vi "HFRR ADV v09.vi"() -> ()   [LabVIEW 2025] (continued)
            n3661 = property on="SPEED OUT:" class="DigNum (strict)"("Caption.Text"=w4886) -> ()  [unwired: 2 in, 2 out]
            n3662 = property on="AIR TEMPERATURE :" class="DigNum (strict)"("Caption.Text"=w4885) -> ()  [unwired: 2 in, 2 out]
            n3663 = property on="HUMIDITY:" class="DigNum (strict)"("Caption.Text"=w4884) -> ()  [unwired: 2 in, 2 out]
            n3664 = property on="EDIT" class="Bool (strict)"("Boolean Text.Text"=w4883) -> ()  [unwired: 2 in, 2 out]
            n3665 = local read "S 79"() -> (w4870:string)
            n3666 = property on="Stroke" class="DigNum (strict)"("Caption.Text"=w4870) -> ()  [unwired: 2 in, 2 out]
          }
          frame #2 {
          }
        }
        n3667 = local write "Lan flag"(10.0 ("Lan flag")) -> ()
      }
      frame Enabled {
      }
    }
    n3668 = Wait (ms)(milliseconds to wait=u32 2000) -> ()  [unwired: 1 out]
    n3669 = local read "Quit"() -> (w4672:bool)
  }
  n3670 = disable-structure shown="Disabled" {
    frame Disabled {
      n3671 = while {
        tunnel: [w4901] -> _
        i -> [w4901]
        stop <- w4900 continue-if-true
        n3672 = Wait (ms)(milliseconds to wait=u32 50) -> ()  [unwired: 1 out]
        n3673 = stacked-sequence {
          frame #0 {
            # "Controls Text color"
            # "Controls BG color"
            n3674 = property on="FILE" class="Str"("Text.Text Colors:Text Color"="SC  Text") -> ()  [unwired: 2 in, 2 out]
            n3675 = property on="Fuel Discription :" class="Str"("Text.Text Colors:Text Color"="SC  Text") -> ()  [unwired: 2 in, 2 out]
            n3676 = property on="tested by" class="Str"("Text.Text Colors:Text Color"="SC  Text") -> ()  [unwired: 2 in, 2 out]
            n3677 = property on="Remarks :" class="Str"("Text.Text Colors:Text Color"="SC  Text") -> ()  [unwired: 2 in, 2 out]
            n3678 = property class="DigNum (strict)"("Numeric Text.Text Colors:BG Color"="NC BG") -> ()  [unwired: 2 in, 2 out]
            n3679 = property class="DigNum (strict)"("Numeric Text.Text Colors:BG Color"="NC BG") -> ()  [unwired: 2 in, 2 out]
            n3680 = property class="DigNum (strict)"("Numeric Text.Text Colors:BG Color"="NC BG") -> ()  [unwired: 2 in, 2 out]
            n3681 = property class="DigNum (strict)"("Numeric Text.Text Colors:BG Color"="NC BG") -> ()  [unwired: 2 in, 2 out]
            n3682 = property class="DigNum (strict)"("Numeric Text.Text Colors:BG Color"="NC BG") -> ()  [unwired: 2 in, 2 out]
            n3683 = property class="DigNum (strict)"("Numeric Text.Text Colors:BG Color"="NC BG") -> ()  [unwired: 2 in, 2 out]
            n3684 = property class="DigNum (strict)"("Numeric Text.Text Colors:BG Color"="NC BG") -> ()  [unwired: 2 in, 2 out]
            n3685 = property class="DigNum (strict)"("Numeric Text.Text Colors:BG Color"="NC BG") -> ()  [unwired: 2 in, 2 out]
            n3686 = property class="DigNum (strict)"("Numeric Text.Text Colors:BG Color"="NC BG") -> ()  [unwired: 2 in, 2 out]
            n3687 = property class="DigNum (strict)"("Numeric Text.Text Colors:BG Color"="NC BG") -> ()  [unwired: 2 in, 2 out]
            n3688 = property class="DigNum (strict)"("Numeric Text.Text Colors:BG Color"="NC BG") -> ()  [unwired: 2 in, 2 out]
            n3689 = property class="DigNum (strict)"("Numeric Text.Text Colors:BG Color"="NC BG") -> ()  [unwired: 2 in, 2 out]
            n3690 = property on="FILE" class="Str"("Text.Text Colors:BG Color"="SC BG 3") -> ()  [unwired: 2 in, 2 out]
            n3691 = property on="Fuel Discription :" class="Str"("Text.Text Colors:BG Color"="SC BG 3") -> ()  [unwired: 2 in, 2 out]
            n3692 = property on="tested by" class="Str"("Text.Text Colors:BG Color"="SC BG 3") -> ()  [unwired: 2 in, 2 out]
            n3693 = property on="Remarks :" class="Str"("Text.Text Colors:BG Color"="SC BG 3") -> ()  [unwired: 2 in, 2 out]
            n3694 = property class="DigNum (strict)"("Numeric Text.Text Colors:Text Color"="NC Text") -> ()  [unwired: 2 in, 2 out]
            n3695 = property class="DigNum (strict)"("Numeric Text.Text Colors:Text Color"="NC Text") -> ()  [unwired: 2 in, 2 out]
            n3696 = property class="DigNum (strict)"("Numeric Text.Text Colors:Text Color"="NC Text") -> ()  [unwired: 2 in, 2 out]
            n3697 = property class="DigNum (strict)"("Numeric Text.Text Colors:Text Color"="NC Text") -> ()  [unwired: 2 in, 2 out]
            n3698 = property class="DigNum (strict)"("Numeric Text.Text Colors:Text Color"="NC Text") -> ()  [unwired: 2 in, 2 out]
            n3699 = property class="DigNum (strict)"("Numeric Text.Text Colors:Text Color"="NC Text") -> ()  [unwired: 2 in, 2 out]
            n3700 = property class="DigNum (strict)"("Numeric Text.Text Colors:Text Color"="NC Text") -> ()  [unwired: 2 in, 2 out]
            n3701 = property class="DigNum (strict)"("Numeric Text.Text Colors:Text Color"="NC Text") -> ()  [unwired: 2 in, 2 out]
            n3702 = property class="DigNum (strict)"("Numeric Text.Text Colors:Text Color"="NC Text") -> ()  [unwired: 2 in, 2 out]
            n3703 = property class="DigNum (strict)"("Numeric Text.Text Colors:Text Color"="NC Text") -> ()  [unwired: 2 in, 2 out]
            n3704 = property class="DigNum (strict)"("Numeric Text.Text Colors:Text Color"="NC Text") -> ()  [unwired: 2 in, 2 out]
            n3705 = property class="DigNum (strict)"("Numeric Text.Text Colors:Text Color"="NC Text") -> ()  [unwired: 2 in, 2 out]
            n3706 = property class="DigNum (strict)"("Numeric Text.Text Colors:Text Color"="NI Text  2") -> ()  [unwired: 2 in, 2 out]
            n3707 = property class="DigNum (strict)"("Numeric Text.Text Colors:Text Color"="NI Text  2") -> ()  [unwired: 2 in, 2 out]
            n3708 = property class="DigNum (strict)"("Numeric Text.Text Colors:Text Color"="NI Text  2") -> ()  [unwired: 2 in, 2 out]
            n3709 = property class="DigNum (strict)"("Numeric Text.Text Colors:Text Color"="NI Text  2") -> ()  [unwired: 2 in, 2 out]
            n3710 = property class="DigNum (strict)"("Numeric Text.Text Colors:Text Color"="NI Text  2") -> ()  [unwired: 2 in, 2 out]
            n3711 = property class="DigNum (strict)"("Numeric Text.Text Colors:Text Color"="NI Text  2") -> ()  [unwired: 2 in, 2 out]
            n3712 = property class="DigNum (strict)"("Numeric Text.Text Colors:Text Color"="NI Text  2") -> ()  [unwired: 2 in, 2 out]
            n3713 = property class="DigNum (strict)"("Numeric Text.Text Colors:Text Color"="NI Text  2") -> ()  [unwired: 2 in, 2 out]
            n3714 = property class="DigNum (strict)"("Numeric Text.Text Colors:Text Color"="NI Text  2") -> ()  [unwired: 2 in, 2 out]
            n3715 = property class="DigNum (strict)"("Numeric Text.Text Colors:Text Color"="NI Text  2") -> ()  [unwired: 2 in, 2 out]
            n3716 = property class="DigNum (strict)"("Numeric Text.Text Colors:Text Color"="NI Text  2") -> ()  [unwired: 2 in, 2 out]
            n3717 = property class="DigNum (strict)"("Numeric Text.Text Colors:Text Color"="NI Text  2") -> ()  [unwired: 2 in, 2 out]
            n3718 = property class="DigNum (strict)"("Numeric Text.Text Colors:Text Color"="NI Text  2") -> ()  [unwired: 2 in, 2 out]
            n3719 = property class="DigNum (strict)"("Numeric Text.Text Colors:Text Color"="NI Text  2") -> ()  [unwired: 2 in, 2 out]
            n3720 = property class="DigNum (strict)"("Numeric Text.Text Colors:Text Color"="NI Text  2") -> ()  [unwired: 2 in, 2 out]
            n3721 = property class="DigNum (strict)"("Numeric Text.Text Colors:Text Color"="NI Text  2") -> ()  [unwired: 2 in, 2 out]
            n3722 = property on="Coefficient Of Friction" class="XYGraph (strict)"("Plot Area:Colors:FG Color"="GFG  2", "Plot Area:Colors:BG Color"="GBG   2") -> ()  [unwired: 2 in, 2 out]
            n3723 = property on="Humidity ( %RH )" class="XYGraph (strict)"("Plot Area:Colors:FG Color"="GFG  2", "Plot Area:Colors:BG Color"="GBG   2") -> ()  [unwired: 2 in, 2 out]
            n3724 = property on="Air Temperature  ( °C )" class="XYGraph (strict)"("Plot Area:Colors:FG Color"="GFG  2", "Plot Area:Colors:BG Color"="GBG   2") -> ()  [unwired: 2 in, 2 out]
            n3725 = property on="Sample Temperature ( °C )" class="XYGraph (strict)"("Plot Area:Colors:FG Color"="GFG  2", "Plot Area:Colors:BG Color"="GBG   2") -> ()  [unwired: 2 in, 2 out]
            n3726 = property class="DigNum (strict)"("Numeric Text.Text Colors:BG Color"="NI BG 2") -> ()  [unwired: 2 in, 2 out]
            n3727 = property class="DigNum (strict)"("Numeric Text.Text Colors:BG Color"="NI BG 2") -> ()  [unwired: 2 in, 2 out]
            n3728 = property class="DigNum (strict)"("Numeric Text.Text Colors:BG Color"="NI BG 2") -> ()  [unwired: 2 in, 2 out]
            n3729 = property class="DigNum (strict)"("Numeric Text.Text Colors:BG Color"="NI BG 2") -> ()  [unwired: 2 in, 2 out]
            n3730 = property class="DigNum (strict)"("Numeric Text.Text Colors:BG Color"="NI BG 2") -> ()  [unwired: 2 in, 2 out]
            n3731 = property class="DigNum (strict)"("Numeric Text.Text Colors:BG Color"="NI BG 2") -> ()  [unwired: 2 in, 2 out]
            n3732 = property class="DigNum (strict)"("Numeric Text.Text Colors:BG Color"="NI BG 2") -> ()  [unwired: 2 in, 2 out]
            n3733 = property class="DigNum (strict)"("Numeric Text.Text Colors:BG Color"="NI BG 2") -> ()  [unwired: 2 in, 2 out]
            n3734 = property class="DigNum (strict)"("Numeric Text.Text Colors:BG Color"="NI BG 2") -> ()  [unwired: 2 in, 2 out]
            n3735 = property class="DigNum (strict)"("Numeric Text.Text Colors:BG Color"="NI BG 2") -> ()  [unwired: 2 in, 2 out]
            n3736 = property class="DigNum (strict)"("Numeric Text.Text Colors:BG Color"="NI BG 2") -> ()  [unwired: 2 in, 2 out]
            n3737 = property class="DigNum (strict)"("Numeric Text.Text Colors:BG Color"="NI BG 2") -> ()  [unwired: 2 in, 2 out]
            n3738 = property class="DigNum (strict)"("Numeric Text.Text Colors:BG Color"="NI BG 2") -> ()  [unwired: 2 in, 2 out]
            n3739 = property class="DigNum (strict)"("Numeric Text.Text Colors:BG Color"="NI BG 2") -> ()  [unwired: 2 in, 2 out]
            n3740 = property class="DigNum (strict)"("Numeric Text.Text Colors:BG Color"="NI BG 2") -> ()  [unwired: 2 in, 2 out]
            n3741 = property class="DigNum (strict)"("Numeric Text.Text Colors:BG Color"="NI BG 2") -> ()  [unwired: 2 in, 2 out]
            n3742 = property class="Bool"("Colors [4]"="Boolean BC T & BG") -> ()  [unwired: 2 in, 2 out]
            n3743 = property on="Save & Continue" class="Bool (strict)"("Colors [4]"="Boolean BC T & BG") -> ()  [unwired: 2 in, 2 out]
            n3744 = property on="Heater Button" class="Bool (strict)"("Colors [4]"="Boolean BC T & BG") -> ()  [unwired: 2 in, 2 out]
            n3745 = property class="Bool"("Colors [4]"="Boolean BC T & BG") -> ()  [unwired: 2 in, 2 out]
            n3746 = property on="Humidity" class="Bool (strict)"("Colors [4]"="Boolean BC T & BG") -> ()  [unwired: 2 in, 2 out]
            n3747 = property class="Bool (strict)"("Colors [4]"="Boolean BC T & BG") -> ()  [unwired: 2 in, 2 out]
            n3748 = property on="RUN" class="Bool (strict)"("Colors [4]"="Boolean BC T & BG") -> ()  [unwired: 2 in, 2 out]
            n3749 = property on="trip1 8" class="Bool (strict)"("Colors [4]"="Boolean BC T & BG") -> ()  [unwired: 2 in, 2 out]
            n3750 = property class="Bool"("Colors [4]"="Boolean BC T & BG") -> ()  [unwired: 2 in, 2 out]
            n3751 = property class="Bool (strict)"("Colors [4]"="Boolean BC T & BG") -> ()  [unwired: 2 in, 2 out]
            n3752 = property on="OPEN 1" class="Bool (strict)"("Colors [4]"="Boolean BC T & BG 2") -> ()  [unwired: 2 in, 2 out]
            n3753 = property on="OPEN 2" class="Bool (strict)"("Colors [4]"="Boolean BC T & BG 2") -> ()  [unwired: 2 in, 2 out]
            n3754 = property on="OPEN 3" class="Bool (strict)"("Colors [4]"="Boolean BC T & BG 2") -> ()  [unwired: 2 in, 2 out]
            n3755 = property on="OPEN 4" class="Bool (strict)"("Colors [4]"="Boolean BC T & BG 2") -> ()  [unwired: 2 in, 2 out]
            n3756 = property on="OPEN" class="Bool (strict)"("Colors [4]"="Boolean BC T & BG 2") -> ()  [unwired: 2 in, 2 out]
            n3757 = property on="rstv2" class="Bool"("Colors [4]"="Boolean BC T & BG 2") -> ()  [unwired: 2 in, 2 out]
            n3758 = property on="RST CP" class="Bool"("Colors [4]"="Boolean BC T & BG 2") -> ()  [unwired: 2 in, 2 out]
            n3759 = property on="RSTV1 3" class="Bool"("Colors [4]"="Boolean BC T & BG 2") -> ()  [unwired: 2 in, 2 out]
            n3760 = property on="RSTV1 2" class="Bool"("Colors [4]"="Boolean BC T & BG 2") -> ()  [unwired: 2 in, 2 out]
          }
          frame #1 {
          }
        }
        n3761 = local read "Quit"() -> (w4900:bool)
      }
    }
    frame Enabled {
    }
  }
  n3762 = while {
    shift-right: [w4918] -> _
    shift-left: _ -> [w4919]
    shift-right: [w4916] -> _
    shift-left: T16 {"Read Heave and Surge"="", "Bytes at Heave Port"=0.0, "Heave and Surge COM Port:"="COM9", "Com Port 2"="COM7", "Residual Due"="", "Heave COM Status 2"=TRUE, "Heave COM Status"=TRUE, "Port 2"=TRUE, "Sway PPR"=6400.0, "Surge PPR"=6400.0, "Heave PPR"=6400.0, "Sway Pitch"=2.0, "Surge Pitch"=3.0, "Heave Pitch"=4.0, "Sway Pulses/mm"=320.0, "Surge Pulses/mm"=1600.0, "Heave Pulses/mm"=1600.0, "inner loop"=0.0, "Read Heave and Surge 2"="", "String 36"="", "Write S"=FALSE, "WriteCC1"=[""], "Heave COM Loop"=0, "LastCom"="", "EXIT"=FALSE, "Error Heave"={"status"=TRUE, "code"=-1073807343, "source"=""}} -> [w4915]
    shift-right: [w4913] -> _
    shift-left: enum16{"init", "MAIN", "Panel Close"}."init" -> [w4914]
    stop <- w4917 stop-if-true
    n3763 = case shown="\"init\"" w4914 {
      tunnel: w4919 -> [w4933 w4948 w5018 w5020]
      tunnel: [w4927 w4966 w5018 w5020] -> w4918
      tunnel: [_ _ TRUE _] -> w4917
      tunnel: [w4923 w4963 w5016 w5019] -> w4916
      tunnel: w4915 -> [w4930 w4947 w5016 w5019]
      tunnel: [enum16{"init", "MAIN", "Panel Close"}."MAIN" w4941 _ _] -> w4913
      frame "init" {
        n3764 = Bundle By Name(cluster=w4930, "Heave and Surge COM Port:"="Humidity :") -> (w4929:T16)
        n3765 = call "Instrument fgv.vi"("Enum"=T26."INIT", "error in (no error) 2"=w4933, "INPUT"=w4929) -> ("error"=w4931:errorcluster, "output"=w4926:T16)  [unwired: 6 in, 1 out]
        n3766 = case shown="No Error" w4931 {
          selector: w4931 -> [w4935 _]
          tunnel: [w4935 w4939] -> w4927
          tunnel: w4926 -> [w4934 w4937]
          tunnel: [w4934 w4936] -> w4924
          frame No Error {
          }
          frame Error {
            n3767 = call "Instrument fgv.vi"("Enum"=T26."ERROR INIT", "INPUT"=w4937) -> ("error"=w4940:errorcluster, "output"=w4936:T16)  [unwired: 7 in, 1 out]
            n3768 = call <vilib>:"Clear Errors.vi"("error in (no error)"=w4940) -> ("error out"=w4939:errorcluster)  [unwired: 5 in, 1 out]
          }
        }
        n3769 = local read "LastCom"() -> (w4922:string)
        n3770 = Unbundle By Name(w4924) -> ("Heave COM Status 2"=→"COM Status" →"Instrument Status":bool, "Error Heave"=→"Error":errorcluster)  [unwired: 1 out]
        n3771 = Bundle By Name(cluster=w4924, "LastCom"=w4922) -> (w4923:T16)
      }
      frame "MAIN" {
        n3772 = Unbundle By Name(w4947) -> ("Com Port 2"=w4968:refnum<visa-resource-name>)
        n3773 = local write "Com Port 4"(w4968) -> ()
        n3774 = local read "Humidity :"() -> (w4945:refnum<visa-resource-name>)
        n3775 = Divide(x="Heave PPR", y="Heave Pitch") -> (x/y=→"Heave Pulses/mm":dbl)
        n3776 = Bundle By Name(cluster=w4947, "Heave and Surge COM Port:"=w4945) -> (w4946:T16)
        n3777 = Equal?(x=w4968, y=w4945) -> (x = y?=w4967:bool)
        n3778 = Divide(x="Sway PPR", y="Sway Pitch") -> (x/y=→"Sway Pulses/mm":dbl)
        n3779 = case shown="False" w4967 {
          tunnel: [w4972 w4989] -> w4966
          tunnel: w4948 -> [w4973 w4995]
          tunnel: w4946 -> [w4971 w4993]
          tunnel: [w4970 w4988] -> w4963
          frame False {
            n3780 = call <vilib>:"Clear Errors.vi"("error in (no error)"=w4973) -> ("error out"=w4969:errorcluster)  [unwired: 5 in, 1 out]
            n3781 = call "Instrument fgv.vi"("Enum"=T26."ERROR INIT", "error in (no error) 2"=w4969, "INPUT"=w4971) -> ("error"=w4975:errorcluster, "output"=w4970:T16)  [unwired: 6 in, 1 out]
            n3782 = call <vilib>:"Clear Errors.vi"("error in (no error)"=w4975) -> ("error out"=w4972:errorcluster)  [unwired: 5 in, 1 out]
          }
          frame True {
            n3783 = call "Instrument fgv.vi"("Enum"=T26."READ", "error in (no error) 2"=w4995, "INPUT"=w4993) -> ("error"=w4994:errorcluster, "output"=w4985:T16)  [unwired: 6 in, 1 out]
            n3784 = Bundle By Name(cluster=w4985, "String 36"="String 11") -> (w4984:T16)
            n3785 = case shown="True" "Write S" {
              selector: "Write S" -> [_ w5015]
              tunnel: w4994 -> [w5008 w5014]
              tunnel: [w5008 w5013] -> w4981
              tunnel: w4984 -> [w5007 w5010]
              tunnel: [w5007 w5009] -> w4980
              frame False {
              }
              frame True {
                n3786 = Not(x=w5015) -> (.not. x?=w5011:bool)
                n3787 = local write "Write S"(w5011) -> ()
                n3788 = call "Instrument fgv.vi"("Enum"=T26."MANUAL WRITE", "error in (no error) 2"=w5014, "INPUT"=w5010) -> ("error"=w5013:errorcluster, "output"=w5009:T16)  [unwired: 6 in, 1 out]
              }
            }
            n3789 = Array Size(array="WriteHumidity") -> (size(s)=w4978:i32)
            n3790 = Greater Than 0?(x=w4978) -> (x > 0?=w4976:bool)
            n3791 = call "Instrument fgv.vi"("Enum"=T26."WRITE", "error in (no error) 2"=w4981, "WriteCC1"="WriteHumidity", "INPUT"=w4980) -> ("error"=w4991:errorcluster, "WriteCC1 2"=w4979:string[], "output"=w4990:T16)  [unwired: 5 in]
            n3792 = case shown="True" w4976 {
              tunnel: w4979 -> [_ w4997]
              frame False {
              }
              frame True {
                n3793 = local write "WriteHumidity"(w4997) -> ()
              }
            }
            n3794 = case shown="Error" w4991 {
              selector: w4991 -> [w4998 w5001]
              tunnel: w4990 -> [w4999 w5006]
              tunnel: [w4999 w5005] -> w4988
              tunnel: [w4998 w5003] -> w4989
              frame No Error {
              }
              frame Error {
                n3795 = call <vilib>:"Clear Errors.vi"("error in (no error)"=w5001) -> ("error out"=w5000:errorcluster)  [unwired: 5 in, 1 out]
                n3796 = call "Instrument fgv.vi"("Enum"=T26."ERROR INIT", "error in (no error) 2"=w5000, "INPUT"=w5006) -> ("error"=w5004:errorcluster, "output"=w5005:T16)  [unwired: 6 in, 1 out]
                n3797 = call <vilib>:"Clear Errors.vi"("error in (no error)"=w5004) -> ("error out"=w5003:errorcluster)  [unwired: 5 in, 1 out]
              }
            }
            n3798 = Unbundle By Name(w4988) -> ("LastCom"=→"LastCom":string, "Read Heave and Surge"=→"Read Humidity":string)
          }
        }
        n3799 = Divide(x="Surge PPR", y="Surge Pitch") -> (x/y=→"Surge Pulses/mm":dbl)
        n3800 = Unbundle By Name(w4963) -> ("Heave COM Status 2"=w4965:bool, "Heave COM Status"=w4964:bool, "Error Heave"=w4961:errorcluster, "Bytes at Heave Port"=→"Bytes at Humidity Port":dbl)
        n3801 = Unbundle By Name(w4961) -> ("status"=→"Humidity Port":bool)
        n3802 = Not(x=w4964) -> (.not. x?=w4949:bool)
        n3803 = local write "Error"(w4961) -> ()
        n3804 = Not(x=w4965) -> (.not. x?=w4950:bool)
        n3805 = local write "Instrument Status"(w4949) -> ()
        n3806 = local write "COM Status"(w4950) -> ()
        n3807 = local read "Quit"() -> (w4942:bool)
        n3808 = Select(t=enum16{"init", "MAIN", "Panel Close"}."Panel Close", s=w4942, f=enum16{"init", "MAIN", "Panel Close"}."MAIN") -> (s? t:f=w4941:enum16{"init", "MAIN", "Panel Close"})
      }
      frame "Panel Close" {
      }
      frame Default {
      }
    }
  }
  n3809 = while {
    stop <- w5046 stop-if-true
    n3810 = local read "Read Humidity"() -> (w5027:string)
    n3811 = call <vilib>:"High Resolution Polling Wait.vi"("seconds to wait"=0.1) -> ()  [unwired: 10 in, 1 out]
    n3812 = Spreadsheet String To Array(delimiter (Tab)=",", format string="", spreadsheet string=w5027, array type (2D Dbl)=string[] []) -> (array=w5041:string[])
    n3813 = for {
      tunnel: w5041 -> [w5051] mode=indexing
      tunnel: string[] ["STATE;", "SET;", "RH;", "T;", "AMB_RH;", "AMB_T;", "PUMP;", "FAN_IN;", "FAN_OUT;", "DEHUM;", "CURRENT;", "STALL;"] -> [w5050] mode=indexing
      tunnel: [w5049] -> w5040 mode=indexing
      n3814 = Match Pattern(string=w5051, regular expression=w5050) -> (after substring=w5049:string)  [unwired: 1 in, 3 out]
    }
    n3815 = Index Array(array=w5040) -> (element #1=→"STATE :":string, element #2=→"SET :":string, element #3=w5029:string, element #4=→"T :":string, element #5=w5026:string, element #6=→"AMB_T :":string, element #7=→"PUMP :":string, element #8=→"FAN_IN :":string, element #9=→"FAN_OUT :":string, element #10=→"DEHUM :":string, element #11=→"CURRENT :":string, element #12=→"STALL :":string)  [unwired: 12 in]
    "RH :" <- w5029
    "AMB_RH :" <- w5026
    n3816 = Fract/Exp String To Number(string=w5029) -> (number=w5021:dbl)  [unwired: 3 in, 1 out]
    n3817 = Fract/Exp String To Number(string=w5026) -> (number=w5025:dbl)  [unwired: 3 in, 1 out]
    n3818 = local write "Ambient Humidity :"(w5025) -> ()
    n3819 = Equal?(x=w5021, y=0.0) -> (x = y?=w5023:bool)
    n3820 = case shown="True" w5023 {
      tunnel: [w5047 w5048] -> w5022
      tunnel: w5021 -> [w5047 _]
      frame False {
        (unwired) 0.0
        "Humidity temp" <- w5047
      }
      frame True {
        n3821 = local read "Humidity temp"() -> (w5048:dbl)
      }
    }
    "RH Numeric:" <- w5022
    n3822 = local read "Quit"() -> (w5046:bool)
  }
  n3823 = disable-structure shown="Disabled" {
    frame Disabled {
      n3824 = while {
        tunnel: [w5285] -> _
        i -> [w5285]
        stop <- w5282 stop-if-true
        n3825 = local read "powstat"() -> (w5283:bool)
        n3826 = case shown="True" w5283 {
          frame False {
          }
          frame True {
            n3827 = local read "RUN"() -> (w5286:bool)
            n3828 = case shown="True" w5286 {
              frame False {
                w5316 = 65.0 ("y")
                n3829 = local read "Set Hz"() -> (w5344:dbl)
                n3830 = local read "NORMAL LOAD"() -> (w5345:dbl)
                n3831 = Multiply(x=w5344, y=60.0) -> (x*y=w5351:dbl)
                n3832 = Multiply(x=1.2 ("y"), y=0.949) -> (x*y=w5320:dbl)
                n3833 = Multiply(x=1.2 ("y"), y=0.8166) -> (x*y=w5324:dbl)
                n3834 = Multiply(x=1.2 ("y"), y=0.851) -> (x*y=w5319:dbl)
                n3835 = local read "FF 2"() -> (w5343:dbl)
                n3836 = Absolute Value(x=w5351) -> (abs(x)=w5349:dbl)
                n3837 = local read "Stroke"() -> (w5318:dbl)
                n3838 = Less?(x=w5318, y=w5324) -> (x < y?=w5321:bool)
                n3839 = In Range and Coerce(upper limit=w5320, x=w5318, lower limit=w5319) -> (In Range?=w5322:bool)  [unwired: 1 out]
                n3840 = case shown="13.." w5343 {
                  tunnel: [1 2 3] -> w5341
                  frame 0..10, Default {
                    # "Normal"
                  }
                  frame 11, 12 {
                  }
                  frame 13.. {
                  }
                }
                "FF STATE" <- w5341
                n3841 = local read "TEMP"() -> (w5304:dbl)
                n3842 = case shown="3601.." w5349 {
                  tunnel: [1 2 3] -> w5347
                  frame 0..3000, Default {
                    # "Normal"
                  }
                  frame 3001..3600 {
                  }
                  frame 3601.. {
                  }
                }
                n3843 = case shown="11.." w5345 {
                  tunnel: [1 3] -> w5346
                  frame 1..10, Default {
                  }
                  frame 11.. {
                  }
                }
                "NL STATE" <- w5346
                n3844 = Multiply(x=1.2 ("y"), y=0.95) -> (x*y=w5334:dbl)
                n3845 = Multiply(x=w5316, y=0.954) -> (x*y=w5308:dbl)
                n3846 = Or(x=w5321, y=w5322) -> (x .or. y?=w5323:bool)
                n3847 = Greater Or Equal?(x=w5318, y=w5334) -> (x >= y?=w5331:bool)
                n3848 = Multiply(x=w5316, y=0.99) -> (x*y=w5305:dbl)
                n3849 = Greater Or Equal?(x=w5304, y=w5305) -> (x >= y?=w5310:bool)
                n3850 = Greater Or Equal?(x=w5304, y=w5308) -> (x >= y?=w5307:bool)
                n3851 = case shown="0, 1, Default" w5318 {
                  tunnel: [1 3] -> w5335
                  frame 0, 1, Default {
                  }
                  frame 2.. {
                  }
                }
                n3852 = case shown="True" w5331 {
                  tunnel: [1 3] -> w5336
                  frame False {
                  }
                  frame True {
                  }
                }
                n3853 = case shown="True" w5323 {
                  tunnel: [1 2] -> w5337
                  frame False {
                  }
                  frame True {
                  }
                }
                n3854 = case shown="..0" w5304 {
                  tunnel: [2 3 3 1] -> w5311
                  frame 61, 62 {
                  }
                  frame 63.. {
                  }
                  frame ..0 {
                  }
                  frame 10..60, Default {
                  }
                }
                n3855 = case shown="True" w5310 {
                  tunnel: [1 3] -> w5312
                  frame False {
                  }
                  frame True {
                  }
                }
                n3856 = Number To Decimal String(number=w5347) -> (decimal integer string=w5348:string)  [unwired: 1 in]
                n3857 = case shown="True" w5307 {
                  tunnel: [1 2] -> w5313
                  frame False {
                  }
                  frame True {
                  }
                }
                n3858 = Number To Decimal String(number=1) -> (decimal integer string=→"Air temp":string)  [unwired: 1 in]
                n3859 = Number To Decimal String(number=w5341) -> (decimal integer string=→"ff_st":string)  [unwired: 1 in]
                n3860 = local write "sp_st"(w5348) -> ()
                n3861 = Number To Decimal String(number=w5346) -> (decimal integer string=→"nl_st":string)  [unwired: 1 in]
                n3862 = Build Array(w5311, w5312, w5313) -> (w5314:i32[])
                n3863 = Build Array(w5335, w5336, w5337) -> (w5338:i32[])
                n3864 = Array Max & Min(array=w5314) -> (max value=w5315:i32)  [unwired: 3 out]
                n3865 = Array Max & Min(array=w5338) -> (max value=w5339:i32)  [unwired: 3 out]
                n3866 = Number To Decimal String(number=w5315) -> (decimal integer string=w5303:string)  [unwired: 1 in]
                n3867 = Number To Decimal String(number=w5339) -> (decimal integer string=→"Stroke Ln 2":string)  [unwired: 1 in]
                n3868 = local write "temp_st"(w5303) -> ()
              }
              frame True {
                w5401 = 65.0 ("y")
                # "Healthy -1\nWarning -2\nError -3"
                n3869 = local read "TEMP"() -> (w5412:dbl)
                n3870 = local read "NORMAL LOAD"() -> (w5416:dbl)
                n3871 = local read "Set Hz"() -> (w5414:dbl)
                n3872 = Multiply(x=1.2 ("y"), y=0.949) -> (x*y=w5396:dbl)
                n3873 = Multiply(x=1.2 ("y"), y=0.8166) -> (x*y=w5392:dbl)
                n3874 = Multiply(x=1.2 ("y"), y=0.851) -> (x*y=w5397:dbl)
                n3875 = Multiply(x=w5401, y=0.954) -> (x*y=w5408:dbl)
                n3876 = Multiply(x=w5401, y=0.99) -> (x*y=w5411:dbl)
                n3877 = Greater Or Equal?(x=w5412, y=w5411) -> (x >= y?=w5406:bool)
                n3878 = Multiply(x=w5414, y=60.0) -> (x*y=w5420:dbl)
                n3879 = Greater Or Equal?(x=w5412, y=w5408) -> (x >= y?=w5409:bool)
                n3880 = local read "FF 2"() -> (w5415:dbl)
                n3881 = local read "Stroke"() -> (w5398:dbl)
                n3882 = Less?(x=w5398, y=w5392) -> (x < y?=w5395:bool)
                n3883 = In Range and Coerce(upper limit=w5396, x=w5398, lower limit=w5397) -> (In Range?=w5394:bool)  [unwired: 1 out]
                n3884 = Absolute Value(x=w5420) -> (abs(x)=w5418:dbl)
                n3885 = case shown="63.." w5412 {
                  tunnel: [2 3 3 1] -> w5405
                  frame 61, 62 {
                  }
                  frame 63.. {
                  }
                  frame ..0 {
                  }
                  frame 10..60, Default {
                  }
                }
                n3886 = case shown="True" w5406 {
                  tunnel: [1 3] -> w5404
                  frame False {
                  }
                  frame True {
                  }
                }
                n3887 = case shown="True" w5409 {
                  tunnel: [1 2] -> w5403
                  frame False {
                  }
                  frame True {
                  }
                }
                n3888 = Multiply(x=1.2 ("y"), y=0.95) -> (x*y=w5382:dbl)
                n3889 = case shown="1..10, Default" w5416 {
                  tunnel: [1 3] -> w5423
                  frame 1..10, Default {
                  }
                  frame 11.. {
                  }
                }
                n3890 = case shown="0..10, Default" w5415 {
                  tunnel: [1 2 3] -> w5422
                  frame 0..10, Default {
                  }
                  frame 11, 12 {
                  }
                  frame 13.. {
                  }
                }
                n3891 = case shown="3601.." w5418 {
                  tunnel: [1 2 3] -> w5417
                  frame 0..3000, Default {
                    # "Normal"
                  }
                  frame 3001..3600 {
                  }
                  frame 3601.. {
                  }
                }
                n3892 = Or(x=w5395, y=w5394) -> (x .or. y?=w5393:bool)
                n3893 = Greater Or Equal?(x=w5398, y=w5382) -> (x >= y?=w5385:bool)
                n3894 = case shown="0, 1, Default" w5398 {
                  tunnel: [1 3] -> w5381
                  frame 0, 1, Default {
                  }
                  frame 2.. {
                  }
                }
                n3895 = case shown="True" w5385 {
                  tunnel: [1 3] -> w5380
                  frame False {
                  }
                  frame True {
                  }
                }
                n3896 = case shown="True" w5393 {
                  tunnel: [1 2] -> w5379
                  frame False {
                  }
                  frame True {
                  }
                }
                n3897 = Build Array(w5405, w5404, w5403) -> (w5402:i32[])
                n3898 = Number To Decimal String(number=w5417) -> (decimal integer string=→"sp_st":string)  [unwired: 1 in]
                n3899 = Array Max & Min(array=w5402) -> (max value=w5399:i32)  [unwired: 3 out]
                "TEMP STATE" <- w5399
                n3900 = Number To Decimal String(number=w5423) -> (decimal integer string=w5426:string)  [unwired: 1 in]
                n3901 = Number To Decimal String(number=w5422) -> (decimal integer string=w5424:string)  [unwired: 1 in]
                n3902 = Number To Decimal String(number=w5399) -> (decimal integer string=→"temp_st":string)  [unwired: 1 in]
                n3903 = Build Array(w5381, w5380, w5379) -> (w5378:i32[])
                n3904 = local write "nl_st"(w5426) -> ()
                n3905 = local write "ff_st"(w5424) -> ()
                n3906 = Number To Decimal String(number=1) -> (decimal integer string=w5421:string)  [unwired: 1 in]
                n3907 = Array Max & Min(array=w5378) -> (max value=w5377:i32)  [unwired: 3 out]
                n3908 = local write "Air temp"(w5421) -> ()
                n3909 = Number To Decimal String(number=w5377) -> (decimal integer string=w5376:string)  [unwired: 1 in]
                n3910 = local write "Stroke Ln 2"(w5376) -> ()
              }
            }
            n3911 = local read "Stroke Ln 2"() -> (w5288:string)
            n3912 = local read "nl_st"() -> (w5294:string)
            n3913 = local read "ff_st"() -> (w5291:string)
            n3914 = local read "sp_st"() -> (w5292:string)
            n3915 = local read "temp_st"() -> (w5293:string)
            n3916 = local read "Air temp"() -> (w5287:string)
            n3917 = Replace Array Subset(array="in", new element #1=w5294, index #1=1 ("index"), new element #2=w5291, index #2=2 ("index"), new element #3=w5293, index #3=3 ("index"), new element #4=w5292, index #4=4 ("index"), new element #5=w5288, index #5=5 ("index"), new element #6=w5287, index #6=6 ("index"), new element #7="Sensor State" ("new element/subarray"), index #7=0 ("index")) -> (→"out":string[])
          }
        }
        n3918 = Wait (ms)(milliseconds to wait=u32 10) -> ()  [unwired: 1 out]
        n3919 = local read "Quit"() -> (w5282:bool)
      }
      n3920 = while {
        stop <- w5257 stop-if-true
        n3921 = local read "run replace"() -> (w5259:bool)
        n3922 = Wait (ms)(milliseconds to wait=u32 100) -> ()  [unwired: 1 out]
        n3923 = Equal?(x="FLAG 2", y=0.0) -> (x = y?=w5260:bool)
        n3924 = case shown="True" w5260 {
          frame False {
          }
          frame True {
            n3925 = local write "FLAG 2"(100.0 ("FLAG 2")) -> ()
            n3926 = call <vilib>:"Read Characters From File.vi"("file path (dialog if empty)"=path "C:/LAB-IQ-NXT/WO 2449 TT.sig", "convert eol? (no:F)"=FALSE ("append to file? (new file:F)")) -> ("character string"=w5263:string)  [unwired: 4 in, 3 out]
            n3927 = call <vilib>:"Read Characters From File.vi"("file path (dialog if empty)"=path "C:/LAB-IQ-NXT/WO 2449 TRH.sig", "convert eol? (no:F)"=FALSE ("append to file? (new file:F)")) -> ("character string"=w5264:string)  [unwired: 4 in, 3 out]
            n3928 = Decimal String To Number(string=w5263) -> (number=w5265:i32)  [unwired: 2 in, 1 out]
            n3929 = local write "Total No. of Tests"(w5265) -> ()
            n3930 = Decimal String To Number(string=w5264) -> (number=w5268:i32)  [unwired: 2 in, 1 out]
            n3931 = local write "SEN.RUN HRS"(w5268) -> ()
          }
        }
        n3932 = case shown="True" w5259 {
          frame False {
          }
          frame True {
            n3933 = Equal?(x="FLAG 4", y=0.0) -> (x = y?=w5272:bool)
            n3934 = case shown="False" w5272 {
              frame False {
                n3935 = Get Date/Time In Seconds() -> (seconds since 1Jan1904=w5278:timestamp)
                n3936 = local read "START 3"() -> (w5276:dbl)
                n3937 = To Double Precision Float(number=w5278) -> (double precision float=w5277:dbl)
                n3938 = Subtract(x=w5277, y=w5276) -> (x-y=→"SENSOR TIME":dbl)
              }
              frame True {
                n3939 = Get Date/Time In Seconds() -> (seconds since 1Jan1904=w5280:timestamp)
                n3940 = local write "FLAG 4"(100.0 ("FLAG")) -> ()
                n3941 = To Double Precision Float(number=w5280) -> (double precision float=→"START 3":dbl)
              }
            }
          }
        }
        n3942 = local read "Quit"() -> (w5257:bool)
      }
      n3943 = while {
        shift-right: [w5057] -> _
        shift-left: _ -> [w5058]
        tunnel: [w5053] -> _
        i -> [w5053]
        stop <- w5052 stop-if-true
        n3944 = Wait (ms)(milliseconds to wait=u32 50 ("Refresh Rate (ms)")) -> ()  [unwired: 1 out]
        n3945 = local read "Json End Flg"() -> (w5054:bool)
        n3946 = Not(x="Upld AR 2") -> ()  [unwired: 1 out]
        n3947 = local read "Upld AR 2"() -> (w5055:bool)
        n3948 = call "Elapsed Time9"("Time Target (s)"="Sen.Upload Rate (s)", "Reset"=FALSE, "Auto Reset"=TRUE) -> ("Time has Elapsed"=w5064:bool)  [unwired: 9 in, 7 out]
        n3949 = Or(x=w5064, y=w5054) -> (x .or. y?=w5060:bool)
        n3950 = case shown="True" w5060 {
          frame False {
          }
          frame True {
            w5156 = "\"SensorName\":\"" ("string")
            w5126 = " \"},{"
            w5151 = "\",\"SensorState\":\""
            w5153 = "\",\"SensorModelNumber\":\"" ("string")
            w5152 = "\",\"SensorRuntimeHours\":\"" ("string")
            n3951 = local read "model num"() -> (w5150:string[])
            n3952 = local read "Sensor name"() -> (w5169:string[])
            n3953 = local read "run"() -> (w5140:string[])
            n3954 = local read "SENSOR TIME"() -> (w5096:dbl)
            n3955 = local read "out"() -> (w5089:string[])
            n3956 = local read "Total No. of Tests"() -> (w5094:dbl)
            n3957 = Select(t=60.0, s="Run test 3", f=3600.0) -> (s? t:f=w5104:dbl)
            n3958 = Index Array(array=w5150, index #1=1 ("index")) -> (element #1=w5149:string, element #2=w5148:string, element #3=w5147:string, element #4=w5146:string, element #5=w5145:string, element #6=w5144:string)  [unwired: 5 in]
            n3959 = Index Array(array=w5140, index #1=1 ("index")) -> (element #1=w5139:string, element #2=w5138:string, element #3=w5137:string, element #4=w5136:string, element #5=w5135:string, element #6=w5134:string)  [unwired: 5 in]
            n3960 = Index Array(array=w5169, index #1=1 ("index")) -> (element #1=w5168:string, element #2=w5167:string, element #3=w5166:string, element #4=w5165:string, element #5=w5155:string, element #6=w5154:string)  [unwired: 5 in]
            n3961 = Index Array(array=w5089, index #1=1 ("index")) -> (element #1=w5121:string, element #2=w5120:string, element #3=w5119:string, element #4=w5118:string, element #5=w5117:string, element #6=w5116:string)  [unwired: 5 in]
            n3962 = local read "SEN.RUN HRS"() -> (w5092:dbl)
            n3963 = Divide(x=w5096, y=w5104) -> (x/y=w5103:dbl)
            n3964 = Increment(x=w5103) -> (x+1=w5099:dbl)
            n3965 = Number To Decimal String(number=w5099) -> (decimal integer string=→"run hrs":string)  [unwired: 1 in]
            n3966 = Divide(x=w5092, y=3600.0 ("f")) -> (x/y=w5087:dbl)
            n3967 = Round To Nearest(number=w5087) -> (nearest integer value=w5085:dbl)
            n3968 = Number To Decimal String(number=w5085) -> (decimal integer string=w5086:string)  [unwired: 1 in]
            n3969 = Number To Decimal String(number=w5094) -> (decimal integer string=w5095:string)  [unwired: 1 in]
            n3970 = local read "Model No"() -> (w5100:string)
            n3971 = local read "UUID"() -> (w5195:string)
            n3972 = local read "Serial No"() -> (w5199:string)
            n3973 = local read "Secret Key"() -> (w5200:string)
            n3974 = Concatenate Strings("\",\"MachineSerialNumber\":\"" ("string"), w5199) -> (w5203:string)
            n3975 = Concatenate Strings("\",\"ModelNumber\":\"" ("string"), w5100) -> (w5101:string)
            n3976 = Concatenate Strings("\",\"MachineRuntimeHours\":\"" ("string"), w5086) -> (w5204:string)
            n3977 = Concatenate Strings("\",\"MachineRuntimeCycles\":\"", w5095) -> (w5197:string)
            n3978 = Concatenate Strings(w5153, w5149) -> (w5183:string)
            n3979 = Concatenate Strings(w5152, w5139) -> (w5184:string)
            n3980 = Concatenate Strings(w5151, w5121) -> (w5182:string)
            n3981 = Concatenate Strings(w5203, w5101, w5204, w5197) -> (w5206:string)
            n3982 = Concatenate Strings(w5153, w5148) -> (w5180:string)
            n3983 = Concatenate Strings(w5152, w5138) -> (w5179:string)
            n3984 = Concatenate Strings(w5151, w5120) -> (w5181:string)
            n3985 = Concatenate Strings(w5153, w5147) -> (w5175:string)
            n3986 = Concatenate Strings(w5152, w5137) -> (w5176:string)
            n3987 = Concatenate Strings(w5151, w5119) -> (w5174:string)
            n3988 = Concatenate Strings(w5153, w5146) -> (w5172:string)
            n3989 = Concatenate Strings(w5152, w5136) -> (w5171:string)
            n3990 = Concatenate Strings(w5151, w5118) -> (w5173:string)
            n3991 = Concatenate Strings(w5183, w5184, w5182) -> (w5185:string)
            n3992 = Concatenate Strings(w5153, w5145) -> (w5162:string)
            n3993 = Concatenate Strings(w5152, w5135) -> (w5163:string)
            n3994 = Concatenate Strings(w5153, w5144) -> (w5159:string)
            n3995 = Concatenate Strings(w5152, w5134) -> (w5158:string)
            n3996 = Concatenate Strings(w5151, w5117) -> (w5161:string)
            n3997 = Concatenate Strings(w5151, w5116) -> (w5160:string)
            n3998 = Concatenate Strings("{\"SecretKey\":\"", w5200, w5206, "\",\"UUID\" : \"", w5195, "\",\"SensorInformation\":", "[{" ("string")) -> (w5133:string)
            n3999 = Concatenate Strings(w5180, w5179, w5181) -> (w5178:string)
            n4000 = Concatenate Strings(w5175, w5176, w5174) -> (w5177:string)
            n4001 = Concatenate Strings(w5172, w5171, w5173) -> (w5170:string)
            n4002 = Concatenate Strings(w5162, w5163, w5161) -> (w5164:string)
            n4003 = Concatenate Strings(w5159, w5158, w5160) -> (w5157:string)
            n4004 = Concatenate Strings(w5156, w5168, w5185, w5126) -> (w5132:string)
            n4005 = Concatenate Strings(w5156, w5167, w5178, w5126) -> (w5131:string)
            n4006 = Concatenate Strings(w5156, w5166, w5177, w5126) -> (w5130:string)
            n4007 = Concatenate Strings(w5156, w5165, w5170, w5126) -> (w5129:string)
            n4008 = Concatenate Strings(w5156, w5155, w5164, w5126) -> (w5128:string)
            n4009 = Concatenate Strings(w5156, w5154, w5157, "\"}" ("string")) -> (w5127:string)
            n4010 = Concatenate Strings(w5133, w5132, w5131, w5130, w5129, w5128, w5127, "]}" ("string")) -> (w5124:string)
            n4011 = local read "SEN.RUN HRS"() -> (w5091:dbl)
            n4012 = disable-structure shown="Disabled" {
              frame Disabled {
                n4013 = local read "state"() -> (w5210:string[])
                n4014 = Delete From Array(array=w5210, index=0) -> (array with subset deleted=w5208:string[])  [unwired: 1 in, 1 out]
                n4015 = for {
                  N: 6 -> [_]
                  tunnel: w5208 -> [w5221] mode=indexing
                  tunnel: [w5220] -> w5207 mode=indexing
                  n4016 = Equal?(x=w5221, y="Warning") -> (x = y?=w5217:bool)
                  n4017 = Equal?(x=w5221, y="Healthy") -> (x = y?=w5214:bool)
                  n4018 = Select(t="2" ("y"), s=w5217, f="3" ("y")) -> (s? t:f=w5212:string)
                  n4019 = Select(t="1" ("y"), s=w5214, f=w5212) -> (s? t:f=w5220:string)
                }
                "state1" <- w5207
              }
              frame Enabled {
              }
            }
            n4020 = stacked-sequence {
              tunnel: w5124 -> [w5232 _ _]
              tunnel: [_ _ w5248] -> _
              frame #0 {
                (unwired) FALSE ("convert eol (F)")
                w5234 = enum16{"start", "end", "current"}."start" ("pos mode (0:2)")
                n4021 = local read "Path"() -> (w5228:path)
                n4022 = Path To String(path=w5228) -> (string=w5240:string)
                n4023 = Concatenate Strings(w5240, "\\", "Sensor File Name") -> (w5241:string)
                n4024 = local write "standard output 2"(" ") -> ()
                n4025 = String To Path(string=w5241) -> (path=w5231:path)
                n4026 = call <vilib>:"Open_Create_Replace File.vi"("advisory dialog? (display:T)"=FALSE, "function (open:0)"=T27."create or replace", "file path"=w5231) -> ("error out"=w5244:errorcluster, "refnum"=w5243:refnum<file>)  [unwired: 5 in, 2 out]
                n4027 = Set File Position(refnum=w5243, from (0:start)=w5234, error in=w5244) -> (refnum out=w5224:refnum<file>, error out=w5223:errorcluster)  [unwired: 1 in]
                n4028 = Write to Binary File(file (use dialog)=w5224, data=" ", error in=w5223, 5:FALSE ("prepend array or string size? (T)")) -> (refnum out=w5235:refnum<file>, error out=w5236:errorcluster)  [unwired: 2 in, 1 out]
                n4029 = Set File Position(offset (in bytes) (0)=w5234, refnum=w5235, error in=w5236) -> (refnum out=w5227:refnum<file>, error out=w5226:errorcluster)  [unwired: 1 in]
                n4030 = Write to Binary File(file (use dialog)=w5227, data=w5232, error in=w5226, 5:FALSE ("prepend array or string size? (T)")) -> (error out=w5230:errorcluster)  [unwired: 2 in, 2 out]
                n4031 = flat-sequence {
                  tunnel: w5231 -> [w5246]
                  tunnel: w5230 -> [_]
                  frame #0 {
                    n4032 = call <vilib>:"Read Characters From File.vi"("file path (dialog if empty)"=w5246) -> ("character string"=→"Sensor Health JSON string":string)  [unwired: 5 in, 3 out]
                  }
                }
                "SinglePoint  2" <- w5232
              }
              frame #1 {
              }
              frame #2 {
                (unwired) "\"Stored\": true" ("string")
                n4033 = call <vilib>:"System Exec.vi"("run minimized? (F)"=TRUE, "wait until completion? (T)"=TRUE, "working directory"=path "C:/LAB-IQ-NXT", "command line"="C:\\LAB-IQ-NXT\\JPostH.bat") -> ("standard error"=→"Respose From Server 2":string, "standard output"=w5251:string)  [unwired: 4 in, 2 out]
                "standard output 2" <- w5251
                n4034 = Match Pattern(string=w5251, regular expression="JSONH Check String") -> (match substring=w5249:string, offset past match=w5248:i32)  [unwired: 1 in, 2 out]
                n4035 = Equal?(x=w5249, y="JSONH Check String") -> (x = y?=→"Upload \nConfirmed 2":bool)
              }
            }
            n4036 = Divide(x=w5091, y=3600.0 ("f")) -> (x/y=w5084:dbl)
            n4037 = local read "run time"() -> (w5141:string[])
            n4038 = Round To Nearest(number=w5084) -> (nearest integer value=w5083:dbl)
            n4039 = Number To Decimal String(number=w5083) -> (decimal integer string=w5082:string)  [unwired: 1 in]
            n4040 = Index Array(array="Sensor Information", index (col) #1=0 ("disabled index (col)"), index (col) #2=1 ("index (col)"), index (col) #3=2 ("index (col)"), index (col) #4=3 ("index (col)")) -> (element #1=→"Sensor name":string[], element #2=→"model num":string[], element #3=→"run time":string[], element #4=→"state":string[])  [unwired: 4 in]
            n4041 = Insert Into Array(array=w5141, index=1, new element #1=w5082, new element #2=w5082, new element #3=w5082, new element #4=w5082, new element #5=w5082, new element #6=w5082) -> (w5106:string[])
            "run" <- w5106
            n4042 = local read "out"() -> (w5088:string[])
            n4043 = local read "Sensor Information"() -> (w5108:string[][])
            n4044 = Replace Array Subset(array=w5108, new element #1=w5106, index (col) #1=2 ("disabled index (col)"), new element #2=w5088, index (col) #2=3 ("index (col)")) -> (w5107:string[][])  [unwired: 2 in]
            n4045 = local write "Sensor Information"(w5107) -> ()
          }
        }
        n4046 = case shown="True" w5055 {
          frame False {
          }
          frame True {
            n4047 = Equal?(x="FLAG", y=0.0) -> (x = y?=w5072:bool)
            n4048 = case shown="False" w5072 {
              frame False {
                n4049 = Get Date/Time In Seconds() -> (seconds since 1Jan1904=w5078:timestamp)
                n4050 = local read "START 2"() -> (w5076:dbl)
                n4051 = To Double Precision Float(number=w5078) -> (double precision float=w5077:dbl)
                n4052 = Subtract(x=w5077, y=w5076) -> (x-y=→"SENSOR TIME  2":dbl)
              }
              frame True {
                n4053 = Get Date/Time In Seconds() -> (seconds since 1Jan1904=w5080:timestamp)
                n4054 = To Double Precision Float(number=w5080) -> (double precision float=→"START 2":dbl)
                n4055 = local write "FLAG"(100.0 ("FLAG")) -> ()
              }
            }
          }
        }
        n4056 = disable-structure shown="Disabled" {
          disable-tunnel: w5058 -> [w5067 _]
          disable-tunnel: [w5066 _] -> w5057
          frame Disabled {
            n4057 = local read "Json St Flg"() -> (w5065:bool)
            n4058 = case shown="True" w5065 {
              tunnel: w5067 -> [w5068 w5070]
              tunnel: [w5068 w5069] -> w5066
              frame False {
              }
              frame True {
                n4059 = Increment(x=w5070) -> (x+1=w5069:dbl)
                "T cycle" <- w5069
                n4060 = local write "Json St Flg"(FALSE ("Json St Flg")) -> ()
              }
            }
          }
          frame Enabled {
          }
        }
        n4061 = local read "Quit"() -> (w5052:bool)
      }
    }
    frame Enabled {
    }
  }
  n4062 = stacked-sequence {
    tunnel: [w5450] -> w30
    frame #0 {
      w5450 = FALSE ("Upload \nConfirmed")
      n4063 = local write "Upload \nConfirmed"(w5450) -> ()
      n4064 = local write "St Str"("") -> ()
    }
  }
  n4065 = disable-structure shown="Disabled" {
    disable-tunnel: w30 -> [w5451 _]
    frame Disabled {
      n4066 = case shown="True" {
        selector: _ -> [_ _]
        tunnel: w5451 -> [_ w5452]
        frame False {
        }
        frame True {
          n4067 = while {
            tunnel: [w5458] -> _
            tunnel: w5452 -> [_]
            i -> [w5458]
            stop <- w5453 stop-if-true
            n4068 = local read "Json End Flg"() -> (w5457:bool)
            n4069 = Wait (ms)(milliseconds to wait=u32 20 ("Refresh Rate (ms)")) -> ()  [unwired: 1 out]
            n4070 = local read "refresh flag"() -> (w5454:bool)
            n4071 = local read "RUN"() -> (w5455:bool)
            n4072 = And(x=w5455, y=w5454) -> (x .and. y?=w5456:bool)
            n4073 = Or(x=w5456, y=w5457) -> (x .or. y?=w5459:bool)
            "AR Led" <- w5459
            n4074 = case shown="True" w5459 {
              frame False {
              }
              frame True {
                w5476 = "\",\""
                n4075 = local read "UUID"() -> (w5474:string)
                n4076 = local write "refresh flag"(FALSE ("refresh flag")) -> ()
                n4077 = local read "time"() -> (w5463:dbl)
                n4078 = Multiply(x=w5463, y=60.0) -> (x*y=w5462:dbl)
                n4079 = Concatenate Strings("UUID\" : \"", w5474, "\"}") -> (w5477:string)
                n4080 = Number To Fractional String(number=w5462, width (-)=i16 10, precision (6)=i16 4) -> (F-format string=w5491:string)  [unwired: 1 in]
                n4081 = Concatenate Strings("{", "\"Time\":\"", w5491, w5476) -> (w5486:string)
                n4082 = stacked-sequence {
                  tunnel: w5476 -> [w5539 w5547 w5554 w5562 w5570 w5579 w5586]
                  tunnel: [w5540 _ _ _ _ _ _] -> w5490
                  tunnel: [_ w5548 _ _ _ _ _] -> w5489
                  tunnel: [_ _ w5555 _ _ _ _] -> w5488
                  tunnel: [_ _ _ w5564 _ _ _] -> w5487
                  tunnel: w5477 -> [_ _ _ _ _ _ w5597]
                  tunnel: [_ _ _ _ _ _ w5596] -> w5473
                  tunnel: [_ _ _ _ _ w5576 _] -> w5472
                  tunnel: [_ _ _ _ w5569 _ _] -> w5471
                  frame #0 {
                    n4083 = local read "NORMAL LOAD"() -> (w5538:dbl)
                    n4084 = Number To Fractional String(number=w5538, width (-)=i16 10, precision (6)=i16 4) -> (F-format string=w5541:string)  [unwired: 1 in]
                    n4085 = Concatenate Strings("NormalLoad\":\"", w5541, w5539) -> (w5540:string)
                  }
                  frame #1 {
                    n4086 = local read "Temp"() -> (w5546:dbl)
                    n4087 = Number To Fractional String(number=w5546, width (-)=i16 10, precision (6)=i16 4) -> (F-format string=w5549:string)  [unwired: 1 in]
                    n4088 = Concatenate Strings("Temperature\":\"", w5549, w5547) -> (w5548:string)
                  }
                  frame #2 {
                    n4089 = local read "cof"() -> (w5552:dbl)
                    n4090 = Number To Fractional String(number=w5552, width (-)=i16 10, precision (6)=i16 4) -> (F-format string=w5556:string)  [unwired: 1 in]
                    n4091 = Concatenate Strings("FrictionalForce\":\"", w5556, w5554) -> (w5555:string)
                  }
                  frame #3 {
                    n4092 = local read "Set Hz"() -> (w5560:dbl)
                    n4093 = Multiply(x=w5560, y=60.0) -> (x*y=w5559:dbl)
                    n4094 = Number To Fractional String(number=w5559, width (-)=i16 10, precision (6)=i16 4) -> (F-format string=w5565:string)  [unwired: 1 in]
                    n4095 = Concatenate Strings("Speed\":\"", w5565, w5562) -> (w5564:string)
                  }
                  frame #4 {
                    n4096 = local read "Stroke Ln"() -> (w5568:dbl)
                    n4097 = Number To Fractional String(number=w5568, width (-)=i16 10, precision (6)=i16 4) -> (F-format string=w5572:string)  [unwired: 1 in]
                    n4098 = Concatenate Strings("LinearDeformation\":\"", w5572, w5570) -> (w5569:string)
                  }
                  frame #5 {
                    n4099 = local read "AIR TEMP"() -> (w5575:dbl)
                    n4100 = local read "Json St Flg"() -> (w5577:bool)
                    n4101 = local read "Json End Flg"() -> (w5578:bool)
                    n4102 = Number To Fractional String(number=w5575, width (-)=i16 10, precision (6)=i16 4) -> (F-format string=w5581:string)  [unwired: 1 in]
                    n4103 = Concatenate Strings("Vibration\":\"", w5581, w5579) -> (w5576:string)
                    n4104 = And(x=w5577, y=w5578) -> ()  [unwired: 1 out]
                  }
                  frame #6 {
                    n4105 = local read "Json End Flg"() -> (w5585:bool)
                    n4106 = Get Date/Time In Seconds() -> (seconds since 1Jan1904=w5593:timestamp)
                    n4107 = local read "Json St Flg"() -> (w5584:bool)
                    n4108 = To Double Precision Float(number=w5593) -> (double precision float=w5592:dbl)
                    n4109 = Subtract(x=w5592, y=2082844800.0) -> (x-y=w5590:dbl)
                    n4110 = Number To Fractional String(number=w5590, width (-)=i16 12, precision (6)=i16 0) -> (F-format string=w5587:string)  [unwired: 1 in]
                    n4111 = case shown="True" w5585 {
                      tunnel: ["" w5600] -> w5594
                      tunnel: w5587 -> [_ w5601]
                      tunnel: w5586 -> [_ w5599]
                      frame False {
                      }
                      frame True {
                        n4112 = local write "Json End Flg"(FALSE ("Json St Flg")) -> ()
                        n4113 = Concatenate Strings("End\": \"", w5601, w5599) -> (w5600:string)
                      }
                    }
                    n4114 = case shown="True" w5584 {
                      tunnel: [w5604 w5607] -> w5595
                      tunnel: w5587 -> [_ w5608]
                      tunnel: w5586 -> [_ w5605]
                      frame False {
                        n4115 = local read "St Str"() -> (w5604:string)
                      }
                      frame True {
                        n4116 = Concatenate Strings("Start\":\"", w5608, w5605) -> (w5607:string)
                        "St Str" <- w5607
                        n4117 = local write "Json St Flg"(FALSE ("Json St Flg")) -> ()
                      }
                    }
                    n4118 = Concatenate Strings(w5595, w5594, w5597) -> (w5596:string)
                  }
                }
                n4119 = local read "FILE"() -> (w5465:string)
                n4120 = Concatenate Strings("\",\"OperatorID\":\"" ("string"), "Operator ID") -> (w5468:string)
                n4121 = Concatenate Strings("\",\"DatasetTitle\":\"" ("string"), w5465) -> (w5467:string)
                n4122 = Concatenate Strings("\",\"SerialNumber\":\"" ("string"), "Serial No") -> (w5497:string)
                n4123 = Concatenate Strings("\",\"ModelNumber\":\"" ("string"), "Model No") -> (w5496:string)
                n4124 = Concatenate Strings(w5497, w5496) -> (w5479:string)
                n4125 = Concatenate Strings("{\"SecretKey\":\"", "Secret Key", w5479, w5468, w5467, "\",\"Samples\":[") -> (w5484:string)
                n4126 = Concatenate Strings(w5486, w5490, w5489, w5488, w5487, w5471, w5472, w5473) -> (w5485:string)
                n4127 = Concatenate Strings(w5484, w5485, "]}") -> (w5483:string)
                n4128 = stacked-sequence {
                  tunnel: w5483 -> [w5512 _ _]
                  tunnel: [_ _ w5529] -> _
                  frame #0 {
                    (unwired) FALSE ("convert eol (F)")
                    w5514 = enum16{"start", "end", "current"}."start" ("pos mode (0:2)")
                    n4129 = Path To String(path="Path") -> (string=w5520:string)
                    n4130 = Concatenate Strings(w5520, "\\", "Data File Name") -> (w5522:string)
                    n4131 = local write "standard output"(" ") -> ()
                    n4132 = String To Path(string=w5522) -> (path=w5511:path)
                    n4133 = call <vilib>:"Open_Create_Replace File.vi"("advisory dialog? (display:T)"=FALSE, "function (open:0)"=T27."create or replace", "file path"=w5511) -> ("error out"=w5525:errorcluster, "refnum"=w5524:refnum<file>)  [unwired: 5 in, 2 out]
                    n4134 = Set File Position(refnum=w5524, from (0:start)=w5514, error in=w5525) -> (refnum out=w5505:refnum<file>, error out=w5504:errorcluster)  [unwired: 1 in]
                    n4135 = Write to Binary File(file (use dialog)=w5505, data=" ", error in=w5504, 5:FALSE ("prepend array or string size? (T)")) -> (refnum out=w5515:refnum<file>, error out=w5516:errorcluster)  [unwired: 2 in, 1 out]
                    n4136 = Set File Position(offset (in bytes) (0)=w5514, refnum=w5515, error in=w5516) -> (refnum out=w5508:refnum<file>, error out=w5507:errorcluster)  [unwired: 1 in]
                    n4137 = Write to Binary File(file (use dialog)=w5508, data=w5512, error in=w5507, 5:FALSE ("prepend array or string size? (T)")) -> (error out=w5510:errorcluster)  [unwired: 2 in, 2 out]
                    n4138 = flat-sequence {
                      tunnel: w5511 -> [w5527]
                      tunnel: w5510 -> [_]
                      frame #0 {
                        n4139 = call <vilib>:"Read Characters From File.vi"("file path (dialog if empty)"=w5527) -> ("character string"=→"JSON string":string)  [unwired: 5 in, 3 out]
                      }
                    }
                    "SinglePoint" <- w5512
                  }
                  frame #1 {
                  }
                  frame #2 {
                    (unwired) "\"Stored\": true" ("string")
                    n4140 = call <vilib>:"System Exec.vi"("run minimized? (F)"=TRUE, "wait until completion? (T)"=TRUE, "working directory"=path "C:/LAB-IQ-NXT", "command line"="C:\\LAB-IQ-NXT\\JPost.bat") -> ("standard error"=→"Respose From Server":string, "standard output"=w5532:string)  [unwired: 4 in, 2 out]
                    "standard output" <- w5532
                    n4141 = Match Pattern(string=w5532, regular expression="JSON Check String") -> (match substring=w5530:string, offset past match=w5529:i32)  [unwired: 1 in, 2 out]
                    n4142 = Equal?(x=w5530, y="JSON Check String") -> (x = y?=→"Upload \nConfirmed":bool)
                  }
                }
              }
            }
            n4143 = local read "Quit"() -> (w5453:bool)
          }
        }
      }
    }
    frame Enabled {
    }
  }
  n4144 = disable-structure shown="Disabled" {
    disable-tunnel: _ -> [w5615 _]
    frame Disabled {
      n4145 = while {
        shift-right: [w5623] -> w5611
        shift-left: _ -> [w5624]
        shift-right: [w5621] -> w5612
        shift-left: errorcluster {"status"=TRUE, "code"=0, "source"="Init"} ("error out") -> [w5622]
        shift-right: [w5619] -> _
        shift-left: "" -> [w5620]
        tunnel: [w5617] -> _
        tunnel: w5615 -> [_]
        i -> [w5617]
        stop <- w5616 stop-if-true
        n4146 = flat-sequence {
          tunnel: [w5625] -> w5618
          frame #0 {
            n4147 = Wait (ms)(milliseconds to wait=10.0 ("Delay")) -> (millisecond timer value=w5625:u32)
          }
        }
        n4148 = case shown="No Error" w5622 {
          selector: w5622 -> [w5658 w5780]
          tunnel: [w5640 w5782] -> w5623
          tunnel: [w5639 w5781] -> w5621
          tunnel: w5624 -> [w5659 w5774]
          tunnel: w5620 -> [w5638 w5773]
          tunnel: [w5637 w5773] -> w5619
          tunnel: w5618 -> [_ _]
          frame No Error {
            n4149 = Concatenate Strings("COMMAND", "\r", "\n") -> (w5649:string)
            n4150 = case shown="True" "Measure" {
              tunnel: w5659 -> [w5685 w5692]
              tunnel: w5658 -> [w5684 w5691]
              tunnel: [w5685 w5690] -> w5657
              tunnel: [w5684 w5689] -> w5636
              tunnel: w5649 -> [_ w5688]
              frame False {
              }
              frame True {
                n4151 = VISA Write(VISA resource name=w5692, write buffer=w5688, error in (no error)=w5691) -> (VISA resource name out=w5690:refnum<visa-resource-name>, error out=w5689:errorcluster)  [unwired: 1 out]
                n4152 = local write "Read String"("") -> ()
                n4153 = local write "Measure"(FALSE) -> ()
              }
            }
